vi "LogIsFull.vi"(8 "Error in (no error)":errorcluster, 11 "LogWriterMock in":refnum<class "LogWriterMock.lvclass">) -> (0 "Error out":errorcluster, 2 "BufferIsFull":bool, 3 "LogWriterMock out":refnum<class "LogWriterMock.lvclass">)   [LabVIEW 2011, in "LogWriterMock.lvclass"]
uses:
  LogWriterMock.lvclass
  LogWriterMock.lvclass/LogWriterMock.ctl
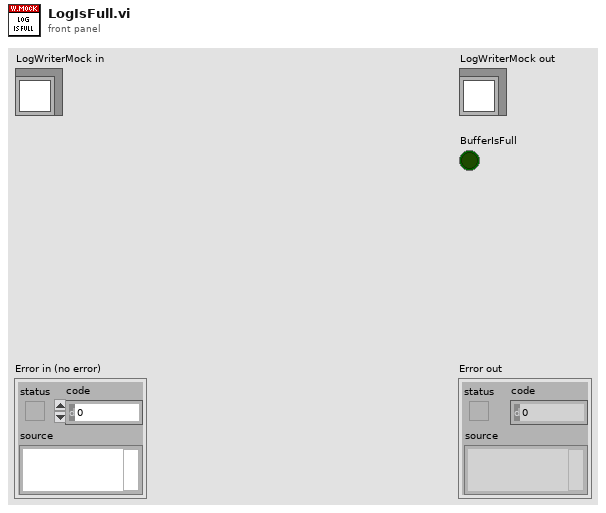
[diagram p1: front panel]
types:
  T1 = typedef "Log.lvclass/Buffer.ctl" = u32
  T2 = typedef "Log.lvclass/LogCluster.ctl" = cluster{"Timestamp":string, "Message":string, "Priority":T3, "PriorityName":string}
  T3 = typedef "Log.lvclass/PrioritiesRing.ctl" = u32
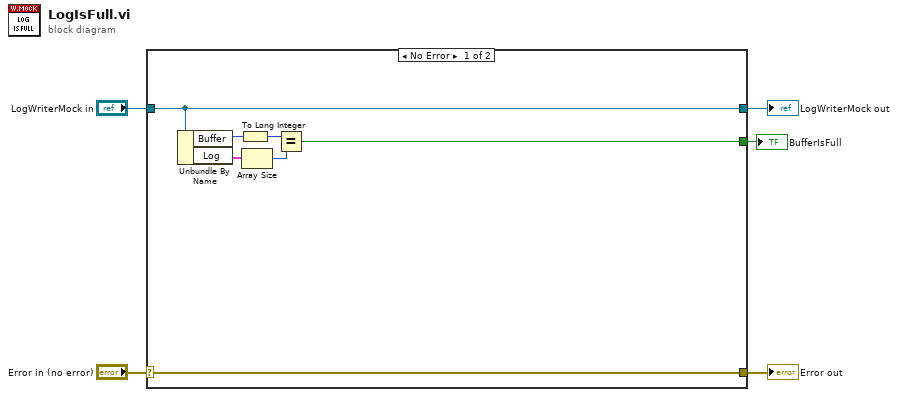
[diagram p0: block diagram]
diagram:
  n1 = case shown="No Error" "Error in (no error)" {
    selector: "Error in (no error)" -> [w12 w14]
    tunnel: [w12 w14] -> w4
    tunnel: [w11 w13] -> w2
    tunnel: "LogWriterMock in" -> [w11 w13]
    tunnel: [w6 _] -> w1
    frame No Error {
      n2 = Unbundle By Name(w11) -> ("Buffer"=w9:T1, "Log"=w10:T2[])
      n3 = To Long Integer(number=w9) -> (32bit integer=w7:i32)
      n4 = Array Size(array=w10) -> (size(s)=w8:i32)
      n5 = Equal?(x=w7, y=w8) -> (x = y?=w6:bool)
    }
    frame Error {
    }
  }
  "Error out" <- w4
  "LogWriterMock out" <- w2
  "BufferIsFull" <- w1
